vi "配置保存.vi"(8 "error in (no error)":errorcluster caption="错误输入（无错误）", 11 "Cleaningcycle 输入":refnum<class "Cleaning cycle.lvclass">) -> (0 "error out":errorcluster caption="错误输出", 3 "Cleaningcycle 输出":refnum<class "Cleaning cycle.lvclass">)   [LabVIEW 2016, in "Cleaning cycle.lvclass"]
uses:
  Cleaning cycle.lvclass
  Cleaning cycle.lvclass/Cleaning cycle.ctl
  <vilib>/Utility/xml.llb/Write to XML File(string).vi
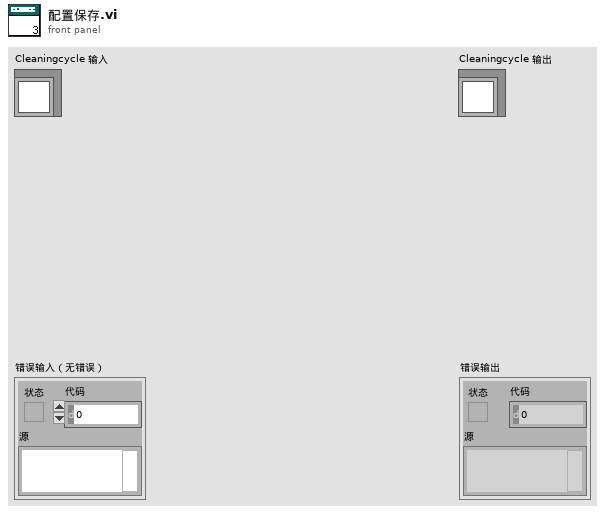
[diagram p1: front panel]
types:
  T1 = typedef "Cleaning cycle.lvclass/State Data.ctl" = cluster{"配置文件路径":path, "简易流程路径":path, "参数列表":cluster{"String":string, "Value":u16}[], "简易流程列表":cluster{"String":string, "Value":u16}[], "配置信息":T2, "命令":cluster{"触发":bool, "周期项":T4}[]}
  T2 = typedef "Cleaning cycle.lvclass/配置信息.ctl" = cluster{"任务列表":T3}
  T3 = typedef "Cleaning cycle.lvclass/任务.ctl" = cluster{"启用":bool, "项":string[][]}
  T4 = typedef "Cleaning cycle.lvclass/周期项.ctl" = cluster{"时":i32, "分":i32, "频次":string, "id":i32, "参数":string, "simpleflowid":i32, "简易流程名称":string}
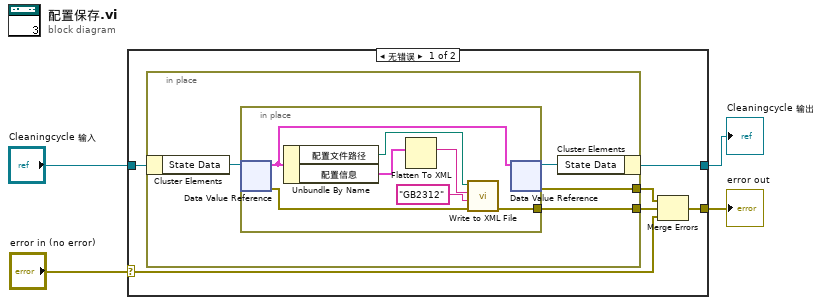
[diagram p0: block diagram]
diagram:
  n1 = case shown="无错误" "error in (no error)" {
    selector: "error in (no error)" -> [w6 w23]
    tunnel: [w5 w23] -> w3
    tunnel: [w9 w22] -> w1
    tunnel: "Cleaningcycle 输入" -> [w10 w22]
    frame No Error {
      n2 = in-place {
        in-place-border: [w12] -> w8
        in-place-border: [w11] -> w7
        n3 = in-place-cluster #1(w10) -> ("State Data"=w14:refnum<data-value>)
        n4 = in-place {
          in-place-border: [w16] -> w11
          n5 = in-place-dvr #2(w14) -> (w18:T1, w17:errorcluster)
          n6 = Unbundle By Name(w18) -> ("配置文件路径"=w15:path, "配置信息"=w19:T2)
          n7 = Flatten To XML(anything=w19) -> (xml string=w21:string)
          n8 = call-poly <vilib>:"Write to XML File.vi"("error in (no error)"=w17, "XML Encoding"="GB2312", "XML Input"=w21, "XML File Path"=w15) -> ("error out"=w16:errorcluster)  [unwired: 5 in, 2 out]
          n9 = in-place-dvr #2(w18) -> (w13:refnum<data-value>, w12:errorcluster)
        }
        n10 = in-place-cluster #1("State Data"=w13) -> (w9:refnum<class "Cleaning cycle.lvclass">)
      }
      n11 = Merge Errors(w8, w7, w6) -> (w5:errorcluster)
    }
    frame Error {
    }
  }
  "error out" <- w3
  "Cleaningcycle 输出" <- w1
